vi "post_artifacts.vi"(8 "error in (no error)":errorcluster, 10 "build_spec_info [] in":T1[](array[typedef]), 11 "lv-builder-default in":refnum<class "lv-builder-default.lvclass">) -> (0 "error out":errorcluster, 2 "build_spec_info [] out":T1[](array[typedef]), 3 "lv-builder-default out":refnum<class "lv-builder-default.lvclass">)   [LabVIEW 2015, in "lv-builder-default.lvclass"]
uses:
  lv-builder-default.lvclass
  lv-build/public/_controls/build_specification.ctl
  lv-build/public/_controls/build_type.ctl
  _controls/configuration.ctl
  _controls/post_action_application.ctl
  _controls/post_action_installer.ctl
  _controls/post_action_zip.ctl
  lv-builder-default.lvlib
  lv-build/lv-build.lvlib
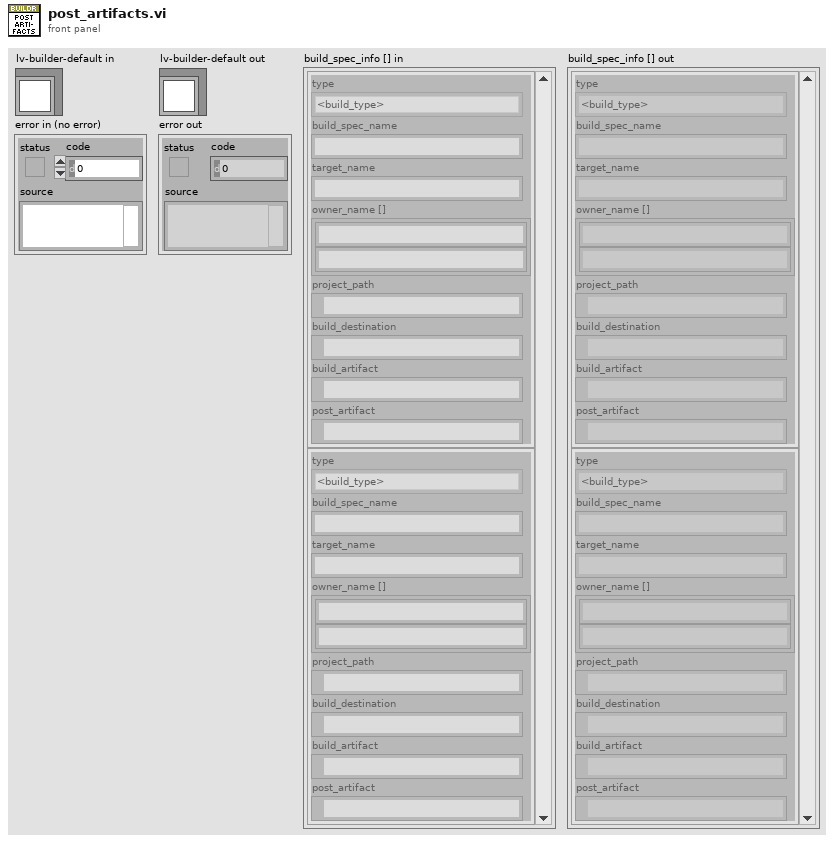
[diagram p1: front panel]
types:
  T1 = typedef "lv-build.lvlib/build_specification.ctl" = cluster{"type":T2, "build_spec_name":string, "target_name":string, "owner_name []":string[], "project_path":path, "build_destination":path, "build_artifact":path, "post_artifact":path}
  T2 = typedef "lv-build.lvlib/build_type.ctl" = enum16{"<build_type>", "application_pc", "application_rt", "installer", "llb", "lvlibp", "zip", "fpga", "<null>"}
  T3 = typedef "lv-builder-default.lvlib/configuration.ctl" = cluster{"project_file":string, "lvlibp_directory":string, "zip_directory":string, "lvlib_directory":string, "update_version_vi":string, "installer_post_file":string, "distribution_folder":string, "dependencies_folder":string, "bin_folder":string, "lvlib_post_action":u16, "installer_post_action":u16, "application_post_action":u16, "zip_post_action":u16}
  T4 = typedef "lv-builder-default.lvlib/post_action_application.ctl" = enum16{"<application_post_action>", "nothing", "zip_application", "<null>"}
  T5 = typedef "lv-builder-default.lvlib/post_action_installer.ctl" = enum16{"<installer_post_action>", "nothing", "create_installer", "zip_installer", "create_installer_file", "<null>"}
  T6 = typedef "lv-builder-default.lvlib/post_action_zip.ctl" = enum16{"<zip_post_action>", "nothing", "move", "extract", "<null>"}
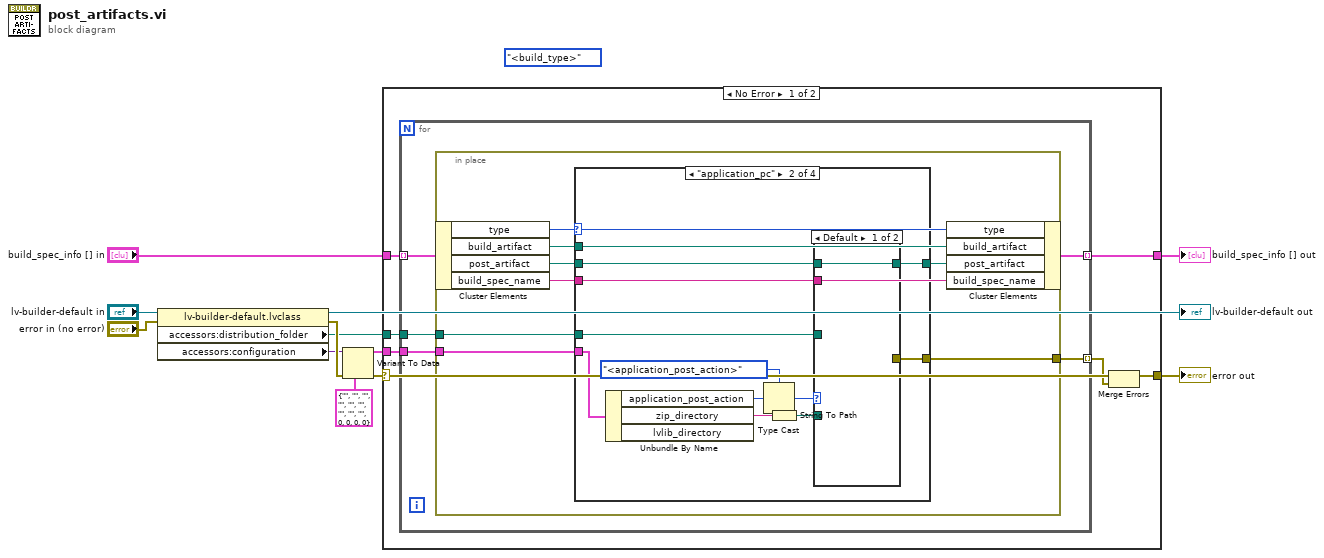
[diagram p0: block diagram]
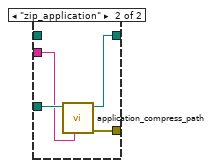
[diagram p3: hidden frame]
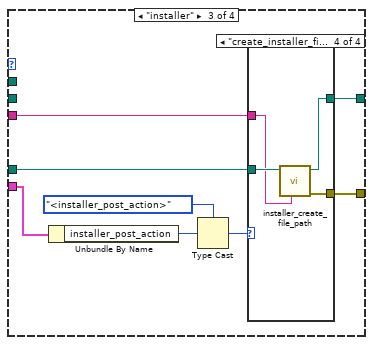
[diagram p4: hidden frame]
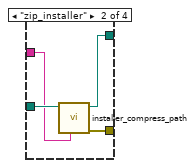
[diagram p6: hidden frame]
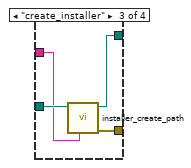
[diagram p7: hidden frame]
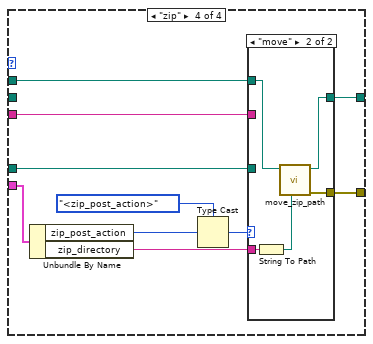
[diagram p8: hidden frame]
diagram:
  (unwired) build_type."<build_type>" ("type")
  n1 = property class="lv-builder-default.lvclass"(reference="lv-builder-default in", error in="error in (no error)") -> (error out=w11:errorcluster, "accessors:distribution_folder"=w3:path, "accessors:configuration"=w4:variant)  [unwired: 1 out]
  n2 = Variant To Data(error in=w11, type=T3 {"project_file"="", "lvlibp_directory"="", "zip_directory"="", "lvlib_directory"="", "update_version_vi"="", "installer_post_file"="", "distribution_folder"="", "dependencies_folder"="", "bin_folder"="", "lvlib_post_action"=0, "installer_post_action"=0, "application_post_action"=0, "zip_post_action"=0} ("configuration"), Variant=w4) -> (data=w5:T3, error out=w2:errorcluster)
  n3 = case shown="No Error" w2 {
    selector: w2 -> [w14 w84]
    tunnel: "build_spec_info [] in" -> [w18 w85]
    tunnel: [w17 w85] -> w9
    tunnel: w5 -> [w16 _]
    tunnel: w3 -> [w15 _]
    tunnel: [w12 w84] -> w1
    frame No Error {
      n4 = for {
        tunnel: w18 -> [w23] mode=indexing
        tunnel: [w22] -> w17 mode=indexing
        tunnel: w16 -> [w21]
        tunnel: w15 -> [w20]
        tunnel: [w19] -> w13 mode=indexing
        n5 = in-place {
          in-place-border: w21 -> [w29]
          in-place-border: w20 -> [w27]
          in-place-border: [w25] -> w19
          n6 = in-place-cluster #1(w23) -> ("type"=w31:T2, "build_artifact"=w28:path, "post_artifact"=w24:path, "build_spec_name"=w26:string)
          n7 = case shown="\"application_pc\"" w31 {
            tunnel: [w32 w35 w50 w72] -> w30
            tunnel: w29 -> [_ w43 w56 w78]
            tunnel: w28 -> [_ _ _ w69]
            tunnel: w27 -> [_ w36 w51 w73]
            tunnel: w26 -> [_ w37 w52 w74]
            tunnel: [_ w34 w49 w71] -> w25
            tunnel: w24 -> [w32 w33 _ _]
            frame Default {
            }
            frame "application_pc" {
              n8 = Unbundle By Name(w43) -> ("application_post_action"=w41:u16, "zip_directory"=w39:string)  [unwired: 1 out]
              n9 = Type Cast(type=post_action_application."<application_post_action>" ("application_post_action"), x=w41) -> (*(type *) &x=w40:T4)
              n10 = String To Path(string=w39) -> (path=w38:path)
              n11 = case shown="Default" w40 {
                tunnel: w38 -> [_ _]
                tunnel: w37 -> [_ w47]
                tunnel: w36 -> [_ w48]
                tunnel: [w44 w46] -> w35
                tunnel: [_ w45] -> w34
                tunnel: w33 -> [w44 _]
                frame Default {
                }
                frame "zip_application" {
                  n12 = call "application_compress_path.vi"("build_spec_name"=w47, "distribution_folder"=w48) -> ("error out"=w45:errorcluster, "path"=w46:path)  [unwired: 8 in]
                }
              }
            }
            frame "installer" {
              n13 = Unbundle By Name(w56) -> ("installer_post_action"=w54:u16)
              n14 = Type Cast(type=post_action_installer."<installer_post_action>" ("installer_post_action"), x=w54) -> (*(type *) &x=w53:T5)
              n15 = case shown="\"create_installer_file\"" w53 {
                tunnel: w52 -> [_ w59 w63 w67]
                tunnel: w51 -> [_ w60 w64 w68]
                tunnel: [_ w58 w62 w66] -> w50
                tunnel: [_ w57 w61 w65] -> w49
                frame Default {
                }
                frame "zip_installer" {
                  n16 = call "installer_compress_path.vi"("build_spec_name"=w59, "distribution_folder"=w60) -> ("error out"=w57:errorcluster, "path"=w58:path)  [unwired: 8 in]
                }
                frame "create_installer" {
                  n17 = call "installer_create_path.vi"("build_spec_name"=w63, "distribution_folder"=w64) -> ("error out"=w61:errorcluster, "path"=w62:path)  [unwired: 8 in]
                }
                frame "create_installer_file" {
                  n18 = call "installer_create_file_path.vi"("build_spec_name"=w67, "distribution_folder"=w68) -> ("error out"=w65:errorcluster, "path"=w66:path)  [unwired: 8 in]
                }
              }
            }
            frame "zip" {
              n19 = Unbundle By Name(w78) -> ("zip_post_action"=w76:u16, "zip_directory"=w70:string)
              n20 = Type Cast(type=post_action_zip."<zip_post_action>" ("zip_post_action"), x=w76) -> (*(type *) &x=w75:T6)
              n21 = case shown="\"move\"" w75 {
                tunnel: w74 -> [_ _]
                tunnel: w73 -> [_ _]
                tunnel: [_ w83] -> w72
                tunnel: [_ w82] -> w71
                tunnel: w70 -> [_ w81]
                tunnel: w69 -> [_ w79]
                frame Default {
                }
                frame "move" {
                  n22 = String To Path(string=w81) -> (path=w80:path)
                  n23 = call "move_zip_path.vi"("zip_move_directory"=w80, "build_artifact"=w79) -> ("error out"=w82:errorcluster, "path"=w83:path)  [unwired: 8 in]
                }
              }
            }
          }
          n24 = in-place-cluster #1("type"=w31, "build_artifact"=w28, "post_artifact"=w30, "build_spec_name"=w26) -> (w22:T1)
        }
      }
      n25 = Merge Errors(w14, w13) -> (w12:errorcluster)
    }
    frame Error {
    }
  }
  "error out" <- w1
  "build_spec_info [] out" <- w9
  "lv-builder-default out" <- "lv-builder-default in"
